vi "Operation Stop.vi"(8 "error in (no error)":errorcluster, 11 "Device Connector in":refnum<class "Device Connector.lvclass">) -> (0 "error out":errorcluster, 3 "Device Connector out":refnum<class "Device Connector.lvclass">)   [LabVIEW 2024, in "Device Connector.lvclass"]
uses:
  Device Connector.lvclass
  Device Connector.lvclass/Device Connector.ctl
  Ancestor Class/Actor/System Actor/System Actor.lvclass
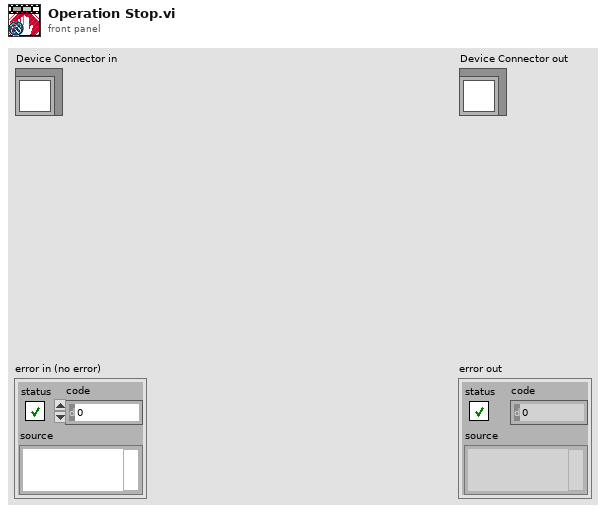
[diagram p1: front panel]
types:
  T1 = typedef "Stop Observer Loop.ctl" = refnum<notifier>
  T2 = typedef "Observer Queue.ctl" = refnum<queue>
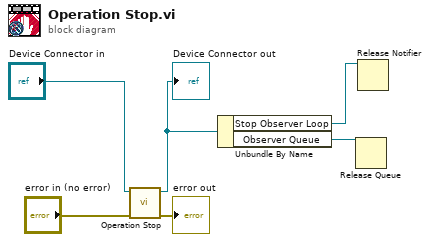
[diagram p0: block diagram]
diagram:
  n1 = call-parent "Operation Stop.vi"("error in (no error)"="error in (no error)", "System Actor in"="Device Connector in") -> ("error out"=→"error out":errorcluster, "System Actor out"=w3:refnum<class "Device Connector.lvclass">)  [unwired: 8 in]
  "Device Connector out" <- w3
  n2 = Unbundle By Name(w3) -> ("Stop Observer Loop"=w2:T1, "Observer Queue"=w1:T2)
  n3 = Release Queue(queue=w1) -> ()  [unwired: 2 in, 3 out]
  n4 = Release Notifier(notifier=w2) -> ()  [unwired: 2 in, 3 out]
